vi "Get Configuration.vi"(11 "Component in":refnum<class "Component.lvclass">) -> (2 "Configuration":refnum<class "Component Configuration.lvclass">, 3 "Component out":refnum<class "Component.lvclass">)   [LabVIEW 2017, in "DSF Core.lvlib" / "Component.lvclass"]
uses:
  Component.lvclass
  Component Configuration/Component Configuration.lvclass
  Component.lvclass/Component.ctl
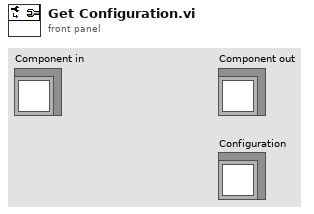
[diagram p1: front panel]
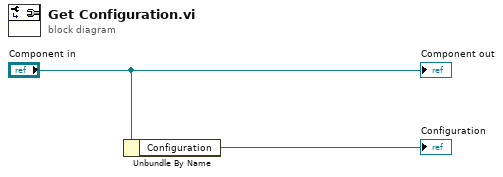
[diagram p0: block diagram]
diagram:
  n1 = Unbundle By Name("Component in") -> ("Configuration"=→"Configuration":refnum<class "Component Configuration.lvclass">)
  "Component out" <- "Component in"
